vi "Globals.vi"() -> ()   [LabVIEW 2013]
uses:
  TCP_IP/TCP_IP.lvclass
  states.ctl
panel:
  in  "cycleContinuously":bool
  in  "state":T1
  in  "Return Data":string
  in  "Log History":string
  in  "Exit Measurement":bool
  in  "connection ID":refnum<k5>
  in  "TCP_IP":refnum<class "TCP_IP.lvclass">
  in  "Return fake test data":bool
  in  "Wait loops":i32
  in  "Log":string
  in  "Restart Network":bool
  in  "Stop":bool
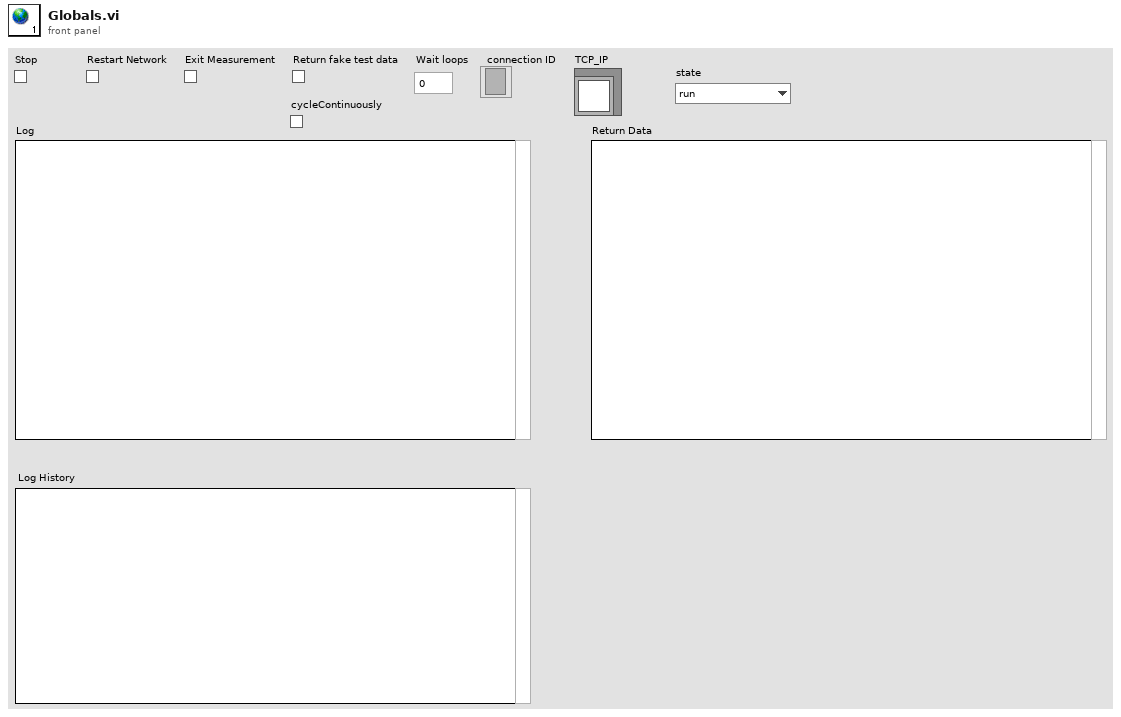
[diagram p1: front panel]
types:
  T1 = typedef "states.ctl" = enum16{"run", "pause", "shutdown gracefully", "halt immediately", "waiting for connection", "waiting for command"}
diagram:
